vi "Parse Core.vi"(0 "SA Path in":refnum<class "SA Abstract Path.lvclass">, 5 "Config Row":string[](array[string]), 11 "error in (no error)":errorcluster) -> (4 "SA Path out":refnum<class "SA Abstract Path.lvclass">, 15 "error out":errorcluster)   [LabVIEW 2023, in "RFFixtureCharact.Public.lvlib" / "SA Abstract Path.lvclass"]
uses:
  SA Abstract Path.lvclass
  SA Abstract Path.lvclass/SA Abstract Path.ctl
  Properties/Write Cal Tone Pin.vi
  Scalar Path/Scalar Path.lvclass
  Common/RFCalAndFixtureCharact.Common.lvlib
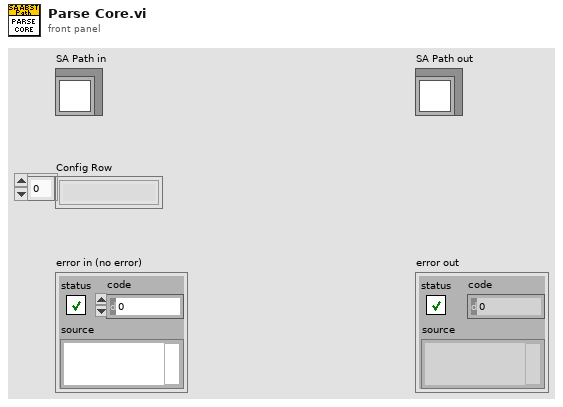
[diagram p1: front panel]
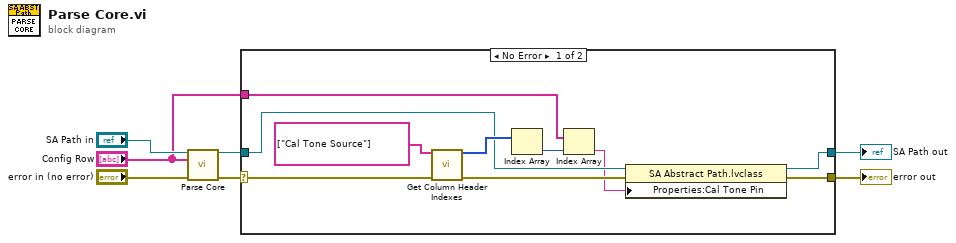
[diagram p0: block diagram]
diagram:
  n1 = call-parent "Parse Core.vi"("Scalar Path in"="SA Path in", "Config Row"="Config Row", "error in (no error)"="error in (no error)") -> ("Scalar Path out"=w5:refnum<class "SA Abstract Path.lvclass">, "error out"=w1:errorcluster)  [unwired: 11 in]
  n2 = case shown="No Error" w1 {
    selector: w1 -> [w8 w19]
    tunnel: w5 -> [w14 w18]
    tunnel: [w12 w19] -> w4
    tunnel: [w11 w18] -> w3
    tunnel: "Config Row" -> [w10 _]
    frame No Error {
      n3 = call "Get Column Header Indexes.vi"("Column Header Names"=string[] ["Cal Tone Source"], "error in"=w8) -> ("Column Header Indices"=w16:i32[], "error out"=w13:errorcluster)  [unwired: 11 in, 1 out]
      n4 = Index Array(array=w16) -> (element=w15:i32)  [unwired: 1 in]
      n5 = Index Array(array=w10, index=w15) -> (element=w9:string)
      n6 = property class="SA Abstract Path.lvclass"(reference=w14, error in=w13, "Properties:Cal Tone Pin"=w9) -> (reference out=w11:refnum<class "SA Abstract Path.lvclass">, error out=w12:errorcluster)
    }
    frame Error {
    }
  }
  "error out" <- w4
  "SA Path out" <- w3
